vi "Read Data.vi"(8 "error in (no error)":errorcluster, 11 "Micron sm Digitizer in":refnum<class "Micron sm Digitizer.lvclass">) -> (0 "error out":errorcluster, 2 "Data":dbl[][](array[numeric]), 3 "Micron sm Digitizer out":refnum<class "Micron sm Digitizer.lvclass">)   [LabVIEW 2024, in "Micron sm Digitizer.lvclass"]
uses:
  Micron sm Digitizer.lvclass
  Micron sm Digitizer.lvclass/Micron sm Digitizer.ctl
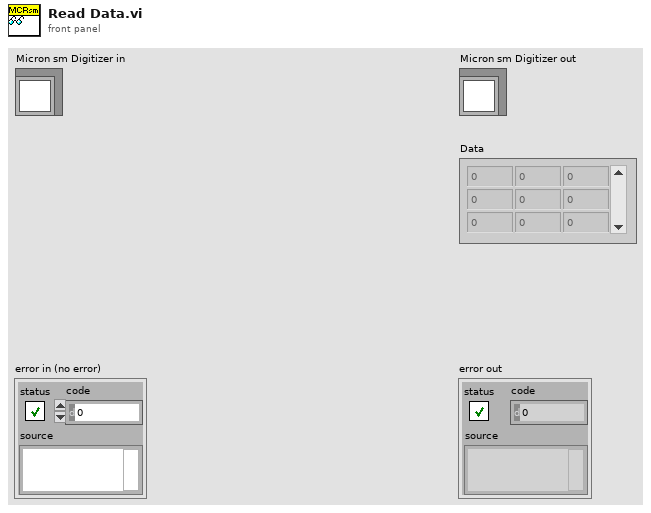
[diagram p1: front panel]
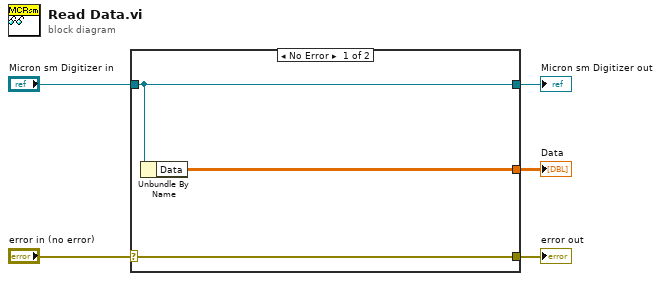
[diagram p0: block diagram]
diagram:
  n1 = case shown="No Error" "error in (no error)" {
    selector: "error in (no error)" -> [w8 w9]
    tunnel: [w8 w9] -> w4
    tunnel: [w7 w10] -> w2
    tunnel: "Micron sm Digitizer in" -> [w7 w10]
    tunnel: [w6 _] -> w1
    frame No Error {
      n2 = Unbundle By Name(w7) -> ("Data"=w6:dbl[][])
    }
    frame Error {
    }
  }
  "error out" <- w4
  "Micron sm Digitizer out" <- w2
  "Data" <- w1
